vi "VII Time Config.vi"(7 "pTimeConfig":T1, 8 "error in (no error)":errorcluster, 9 "I2CIndex":i32, 10 "DevIndex":i32, 11 "DevType":i32) -> (0 "error out":errorcluster, 3 "function return":i32, 5 "pTimeConfig out":T1)   [LabVIEW 2011, in "ControlI2C.lvlib"]
doc: "int __stdcall VII_TimeConfig(int DevType, int DevIndex, int I2CIndex, PVII_TIME_CONFIG pTimeConfig);"
uses:
  ControlI2C.lvlib
  1234/Ginkgo_Driver.dll
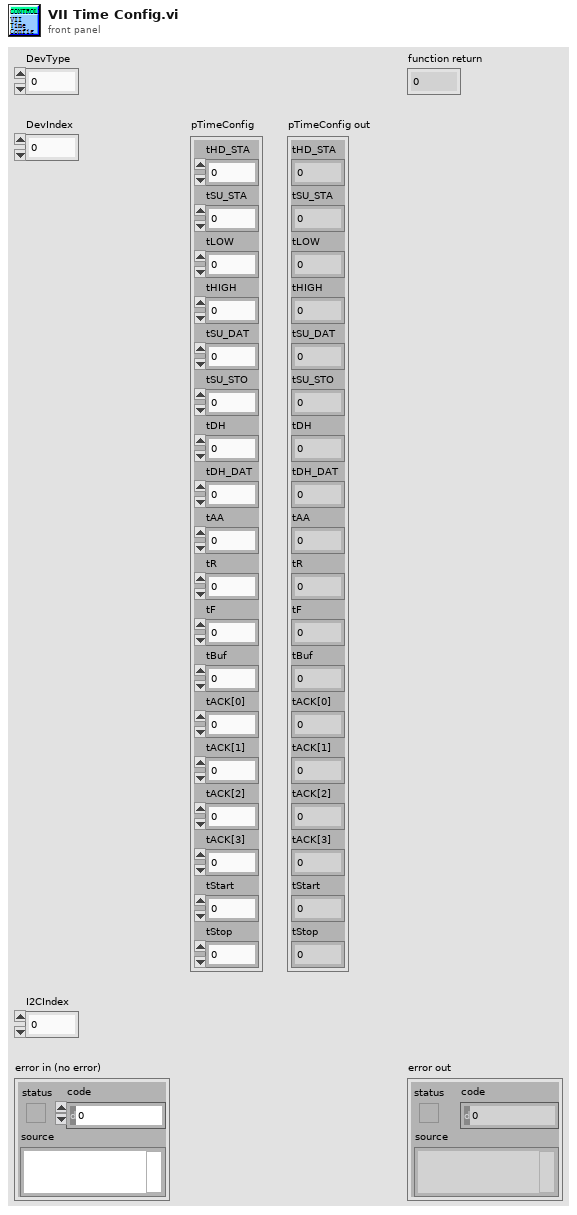
[diagram p1: front panel]
types:
  T1 = cluster{"tHD_STA":u16, "tSU_STA":u16, "tLOW":u16, "tHIGH":u16, "tSU_DAT":u16, "tSU_STO":u16, "tDH":u16, "tDH_DAT":u16, "tAA":u16, "tR":u16, "tF":u16, "tBuf":u16, "tACK[0]":u8, "tACK[1]":u8, "tACK[2]":u8, "tACK[3]":u8, "tStart":u16, "tStop":u16}
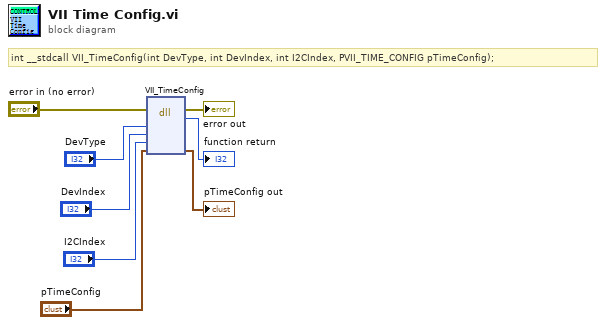
[diagram p0: block diagram]
diagram:
  # "int __stdcall VII_TimeConfig(int DevType, int DevIndex, int I2CIndex, PVII_TIME_CONFIG pTimeConfig);"
  n1 = dll-call lib="E:/Project/vt_ginkgo/truck/Ginkgo Driver/vs2010/Ginkgo_USB-I2C&SPI&CAN_API_v2.0.3.3/lib/labview_32bit/1234/Ginkgo_Driver.*" fn="VII_TimeConfig"(error in="error in (no error)", "DevType"="DevType", "DevIndex"="DevIndex", "I2CIndex"="I2CIndex", "pTimeConfig"="pTimeConfig") -> (error out=→"error out":errorcluster, →"function return":i32, "pTimeConfig"=→"pTimeConfig out":T1)  [unwired: 5 in, 1 out]
